vi "LN2.GetPrivateEvents.vi"(8 "error in (no error)":errorcluster, 11 "Instrument.LN2 in":refnum<class "Instrument.LN2.lvclass">) -> (0 "error out":errorcluster, 2 "PrivateEvents":T1, 3 "Instrument.LN2 out":refnum<class "Instrument.LN2.lvclass">)   [LabVIEW 2019, in "Instrument.LN2.lvclass"]
uses:
  Instrument.LN2.lvclass
  Typedefs/PrivateEvents--Cluster.ctl
  Typedefs/PrivateEvents--Instrument.MessageToProcess.ctl
  <userlib>/LevyLab/Instrument Framework/SMOs/RemoteControl/Typedefs/Message--Cluster.ctl
  Instrument.LN2.lvclass/Instrument.LN2.ctl
  <userlib>/LevyLab/Instrument Framework/SMOs/RemoteControl/RemoteControl.lvclass
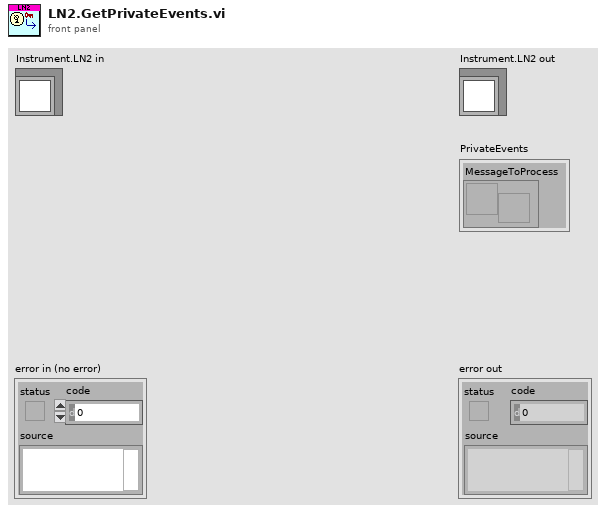
[diagram p1: front panel]
types:
  T1 = typedef "Instrument.LN2.lvclass/PrivateEvents--Cluster.ctl" = cluster{"MessageToProcess":refnum<user-event>}
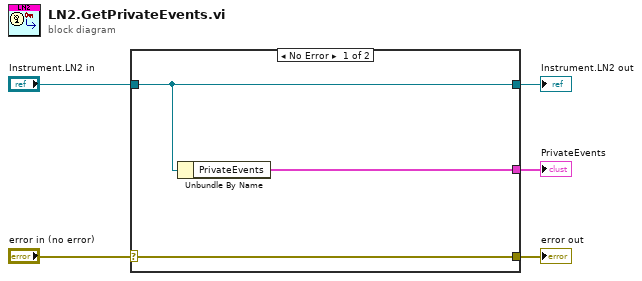
[diagram p0: block diagram]
diagram:
  n1 = case shown="No Error" "error in (no error)" {
    selector: "error in (no error)" -> [w8 w9]
    tunnel: [w8 w9] -> w4
    tunnel: [w7 w10] -> w2
    tunnel: "Instrument.LN2 in" -> [w7 w10]
    tunnel: [w6 _] -> w1
    frame No Error {
      n2 = Unbundle By Name(w7) -> ("PrivateEvents"=w6:T1)
    }
    frame Error {
    }
  }
  "error out" <- w4
  "Instrument.LN2 out" <- w2
  "PrivateEvents" <- w1
